vi "Frontend FPP_vdp_Ian_modified.vi"() -> ()   [LabVIEW 2016]
panel:
  in  "Gate 2":T1={"Gate Start"=0.0, "Gate Stop"=2.0, "Gate Step (linear only)"=1.0, "Gate Compliance"=0.0001, "Gate PComp"=0.0, "Range mode"=0, "Range"=6} {"Range" max=11 scale=0.0..11.0; "Range mode" items=["Auto", "Limited", "Fixed"]; "Gate PComp" format="%^.2e"; "Gate Compliance" format="%^.2e"; "Gate Step (linear only)" format="%^.4e"; "Gate Stop" format="%^.4e"; "Gate Start" format="%^.4e"}
  in  "Drain":T2={"Drain Start"=0.0, "Drain Stop"=2.0, "Drain Compliance"=0.0001, "Drain Step"=1.0, "Drain PComp"=0.0, "Range mode"=0, "Range"=6} {"Range" max=11 scale=0.0..11.0; "Range mode" items=["Auto", "Limited", "Fixed"]; "Drain PComp" format="%^.2e"; "Drain Step" format="%^.4e"; "Drain Compliance" format="%^.2e"; "Drain Stop" format="%^.4e"; "Drain Start" format="%^.4e"}
  in  "Gate":T3={"Gate Start"=0.0, "Gate Stop"=2.0, "Gate Step"=1.0, "Gate Compliance"=0.0001, "Gate PComp"=0.0, "Range mode"=0, "Range"=6} {"Range" max=11 scale=0.0..11.0; "Range mode" items=["Auto", "Limited", "Fixed"]; "Gate PComp" format="%^.2e"; "Gate Compliance" format="%^.2e"; "Gate Step" format="%^.4e"; "Gate Stop" format="%^.4e"; "Gate Start" format="%^.4e"}
  in  "Drain 2":T4={"Drain Start"=0.0, "Drain Stop"=2.0, "Drain Compliance"=0.0001, "Drain Step (linear only)"=1.0, "Drain PComp"=0.0, "Range mode"=0, "Range"=6} {"Range" max=11 scale=0.0..11.0; "Range mode" items=["Auto", "Limited", "Fixed"]; "Drain PComp" format="%^.2e"; "Drain Step (linear only)" format="%^.4e"; "Drain Compliance" format="%^.2e"; "Drain Stop" format="%^.4e"; "Drain Start" format="%^.4e"}
  in  "Timings":T5={"integration time"=0, "Short/Long integration time"=0.00064, "hold time (sec)"=0.0, "delay time (sec)"=0.0, "Step Time (0 disables)"=0.0, "sweep method"=0, "Pulse period"=0.005, "Base voltage"=0.0, "Pulse width"=0.0005} {"Pulse width" min=0.0005 max=0.1 step=0.0001 format="%.4f"; "Base voltage" format="%^.4e"; "Pulse period" min=0.005 max=1.0 step=0.0001 format="%.4f"; "sweep method" items=["Continuous", "Pulsed"]; "Step Time (0 disables)" format="%.2f"; "delay time (sec)" format="%.4f"; "hold time (sec)" format="%.4f"; "Short/Long integration time" format="%^.0e"; "integration time" scale=0.0..2.0}
  in  "Panel controls":T6={"Emergency Stop"=refnum, "OutputGraph Max"=1e-05, "Text/Graph (text=false)"=FALSE} {"OutputGraph Max" format="%.2e"}
  in  "Panel Controls":T7={"Emergency Stop"=refnum, "TransGraph Max"=1e-05, "Text/Graph (text=false)"=FALSE} {"TransGraph Max" format="%.2e"}
  in  "Tab Control":enum32{"Characteristics", "Other parameters"}(tab)
  in  "Van der Pauw":bool
  out "XY Graph 2":cluster{"Y data in":dbl[], "X data in":dbl[]}[](graph)
  in  "Integration time (long)":dbl=0.32 min=0.04 max=2.0 step=0.02 format="%.2f"
  in  "Integration time (short)":dbl=0.00064 min=8e-05 max=0.00192 step=8e-05 format="%^.0e"
  in  "Drain Range":u8(slide)=6 max=11 scale=0.0..11.0
  in  "Drain Range mode":u16(ring) items=["Auto", "Limited", "Fixed"]
  in  "Gate Range":u8(slide)=6 max=11 scale=0.0..11.0
  in  "Gate Range mode":u16(ring) items=["Auto", "Limited", "Fixed"]
  in  "Sampling mode":u32(slide) scale=0.0..4.0
  in  "Number of Samples":i32=500 min=0 step=1
  in  "Time":dbl=240.0 min=0.0 format="%.2f"
  in  "Drain":dbl=-10.0 min=-100.0 max=100.0 format="%.2f"
  in  "Gate":dbl=-60.0 min=-100.0 max=100.0 format="%.2f"
  in  "sweep method":u16(ring) items=["Continuous", "Pulsed"]
  out "Id":dbl format="%.2e"
  out "Ig":dbl format="%.2e"
  in  "Sweep Start":bool caption="Sweep start"
  in  "Interrupt run":bool
  in  "Running":bool
  out "Path":path
  in  "integration time":u32(slide)=1 max=2 step=1 scale=0.0..2.0
  in  "sweep mode":u16(ring)=1 items=["Single", "Double"]
  in  "Transfer Start":bool
  in  "Output Start":bool
  in  "Drain: Step":dbl=-0.1 min=-100.0 max=100.0 format="%.2f"
  in  "Drain: Stop":dbl=-1.0 min=-100.0 max=100.0 format="%.2f"
  in  "Drain:Start":dbl=1.0 min=-100.0 max=100.0 format="%.2f"
  in  "Gate: Step":dbl min=-100.0 max=100.0 format="%.2f"
  in  "Gate: Stop":dbl min=-100.0 max=100.0 format="%.2f"
  in  "Gate: Start":dbl min=-100.0 max=100.0 format="%.2f"
  out "XY Graph":cluster{"Y data in":dbl[], "X data in":dbl[]}[](graph)
  in  "Drain: Compliance":dbl=0.001 min=1e-12 max=0.02 format="%.8f"
  in  "Gate: Compliance":dbl=0.001 min=1e-12 max=0.02 format="%.8f"
  in  "Drain: Step":dbl=-5.0 min=-100.0 max=100.0 format="%.2f"
  in  "Drain: Stop":dbl=-10.0 min=-100.0 max=100.0 format="%.2f"
  in  "Drain:Start":dbl=-5.0 min=-100.0 max=100.0 format="%.2f"
  in  "Gate: Step":dbl=-1.0 min=-100.0 max=100.0 format="%.2f"
  in  "Gate: Stop":dbl=-60.0 min=-100.0 max=100.0 format="%.2f"
  in  "Gate: Start":dbl=10.0 min=-100.0 max=100.0 format="%.2f"
  out "Vp_2":dbl format="%.2e"
  out "Vp_1":dbl format="%.2e"
  out "Delta V":dbl format="%.2e"
  out "Conductivity (S/cm)":dbl format="%.2e"
  in  "Thickness (m)":dbl=4e-08 min=1e-09 max=100.0 format="%.2e"
  in  "Hall Bar Channel Length  (L in m)":dbl=2e-05 format="%#_13g"
  in  "Hall Bar Channel Width (W in m)":dbl=4e-05 format="%#_13g"
  in  "Pulse width":dbl=0.0005 min=0.0005 max=0.1 step=0.0001 format="%.4f"
  in  "Base voltage":dbl min=-100.0 max=100.0 format="%.2f"
  in  "Pulse period":dbl=0.005 min=0.005 max=1.0 step=0.0001 format="%.4f"
  in  "Drain Power Compliance":dbl min=0.0 max=1.0 format="%.2f"
  in  "Gate Power\nCompliance":dbl min=0.0 max=1.0 format="%.2f"
  in  "OutputGraph Max":dbl=1e-05 format="%.2e"
  in  "TransGraph Max":dbl=1e-05 format="%.2e"
  in  "SPA Display":bool
  in  "Step delay /s":dbl min=0.0 max=1.0 format="%.2f"
  in  "hold time /s":dbl min=0.0 max=655.35 step=0.01 format="%.2f"
  in  "delay time /s":dbl min=0.0 max=65.535 step=0.0001 format="%.2f"
  in  "Decimal places in header":i8=1
  out "error out":errorcluster
  # "Transfer Characteristics"
  # "Stress Measurements"
  # "V"
  # "V"
  # "V"
  # "Gate"
  # "V"
  # "V"
  # "V"
  # "V"
  # "Drain"
  # "V"
  # "Output Characteristics"
  # "s"
  # "V"
  # "V"
  # "V"
  # "Gate"
  # "V"
  # "V"
  # "Drain"
  # "V"
  # "For Four Point Probe measurements ONLY!"
  # "SMU1 = Probe 1\nSMU2 = Drain\nSMU3 = Gate\nSMU4 = Probe 2\nVSU1 = Source"
  # "A"
  # "A"
  # "Vp1"
  # "Vp2"
  # "s"
  # "Pulsed mode settings"
  # "s"
  # "NOTE - THIS OVERRIDES THE COMPLIANCE VALUES!"
  # "A"
  # "A"
  # "Enter max power in Watts (max 1W)"
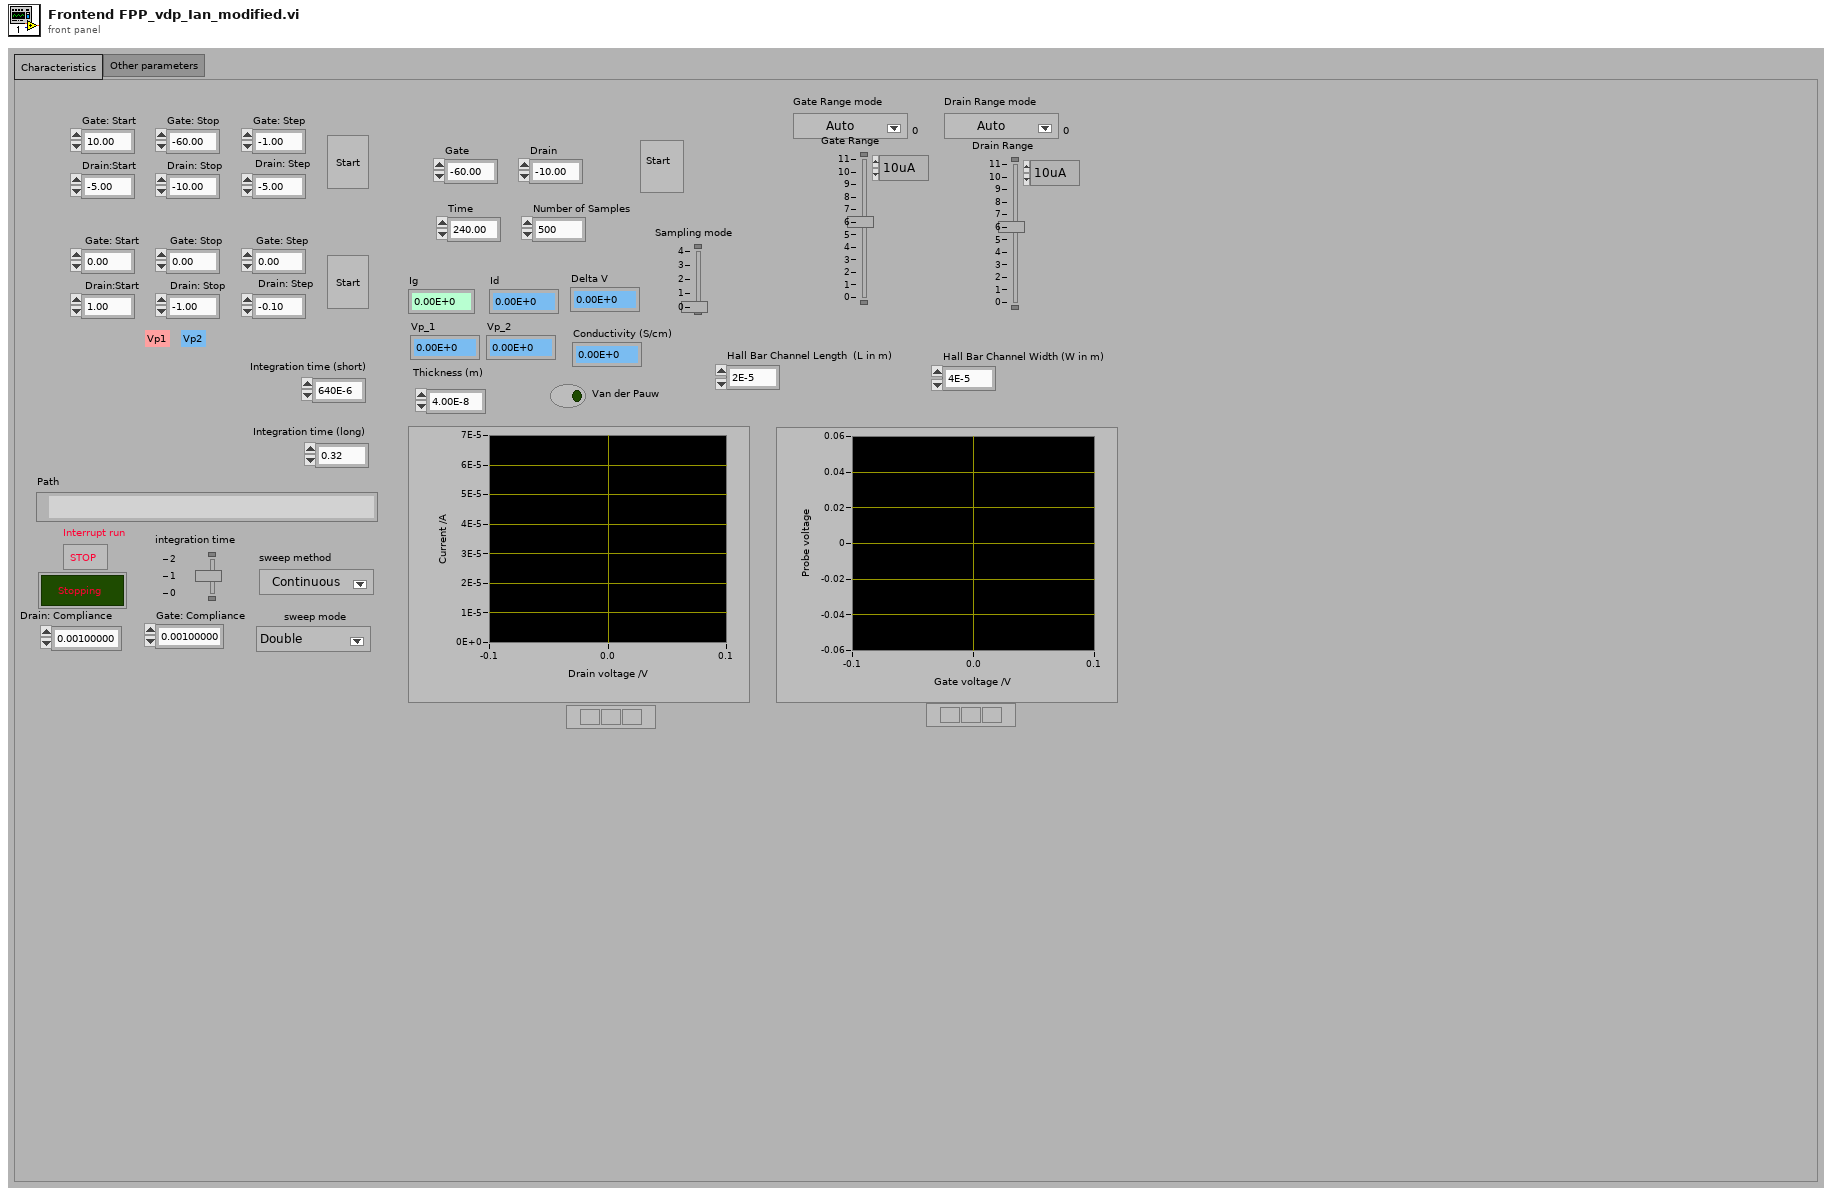
[diagram p1: front panel]
types:
  T1 = cluster{"Gate Start":dbl, "Gate Stop":dbl, "Gate Step (linear only)":dbl, "Gate Compliance":dbl, "Gate PComp":dbl, "Range mode":u16, "Range":u8}
  T2 = cluster{"Drain Start":dbl, "Drain Stop":dbl, "Drain Compliance":dbl, "Drain Step":dbl, "Drain PComp":dbl, "Range mode":u16, "Range":u8}
  T3 = cluster{"Gate Start":dbl, "Gate Stop":dbl, "Gate Step":dbl, "Gate Compliance":dbl, "Gate PComp":dbl, "Range mode":u16, "Range":u8}
  T4 = cluster{"Drain Start":dbl, "Drain Stop":dbl, "Drain Compliance":dbl, "Drain Step (linear only)":dbl, "Drain PComp":dbl, "Range mode":u16, "Range":u8}
  T5 = cluster{"integration time":u32, "Short/Long integration time":dbl, "hold time (sec)":dbl, "delay time (sec)":dbl, "Step Time (0 disables)":dbl, "sweep method":u16, "Pulse period":dbl, "Base voltage":dbl, "Pulse width":dbl}
  T6 = cluster{"Emergency Stop":refnum<vi>, "OutputGraph Max":dbl, "Text/Graph (text=false)":bool}
  T7 = cluster{"Emergency Stop":refnum<vi>, "TransGraph Max":dbl, "Text/Graph (text=false)":bool}
  T8 = cluster{"V2 Start":dbl, "V2 Step":dbl, "Number of points":i32}
  T9 = enum16{"open", "replace", "create", "open or create", "replace or create", "replace or create with confirmation"}
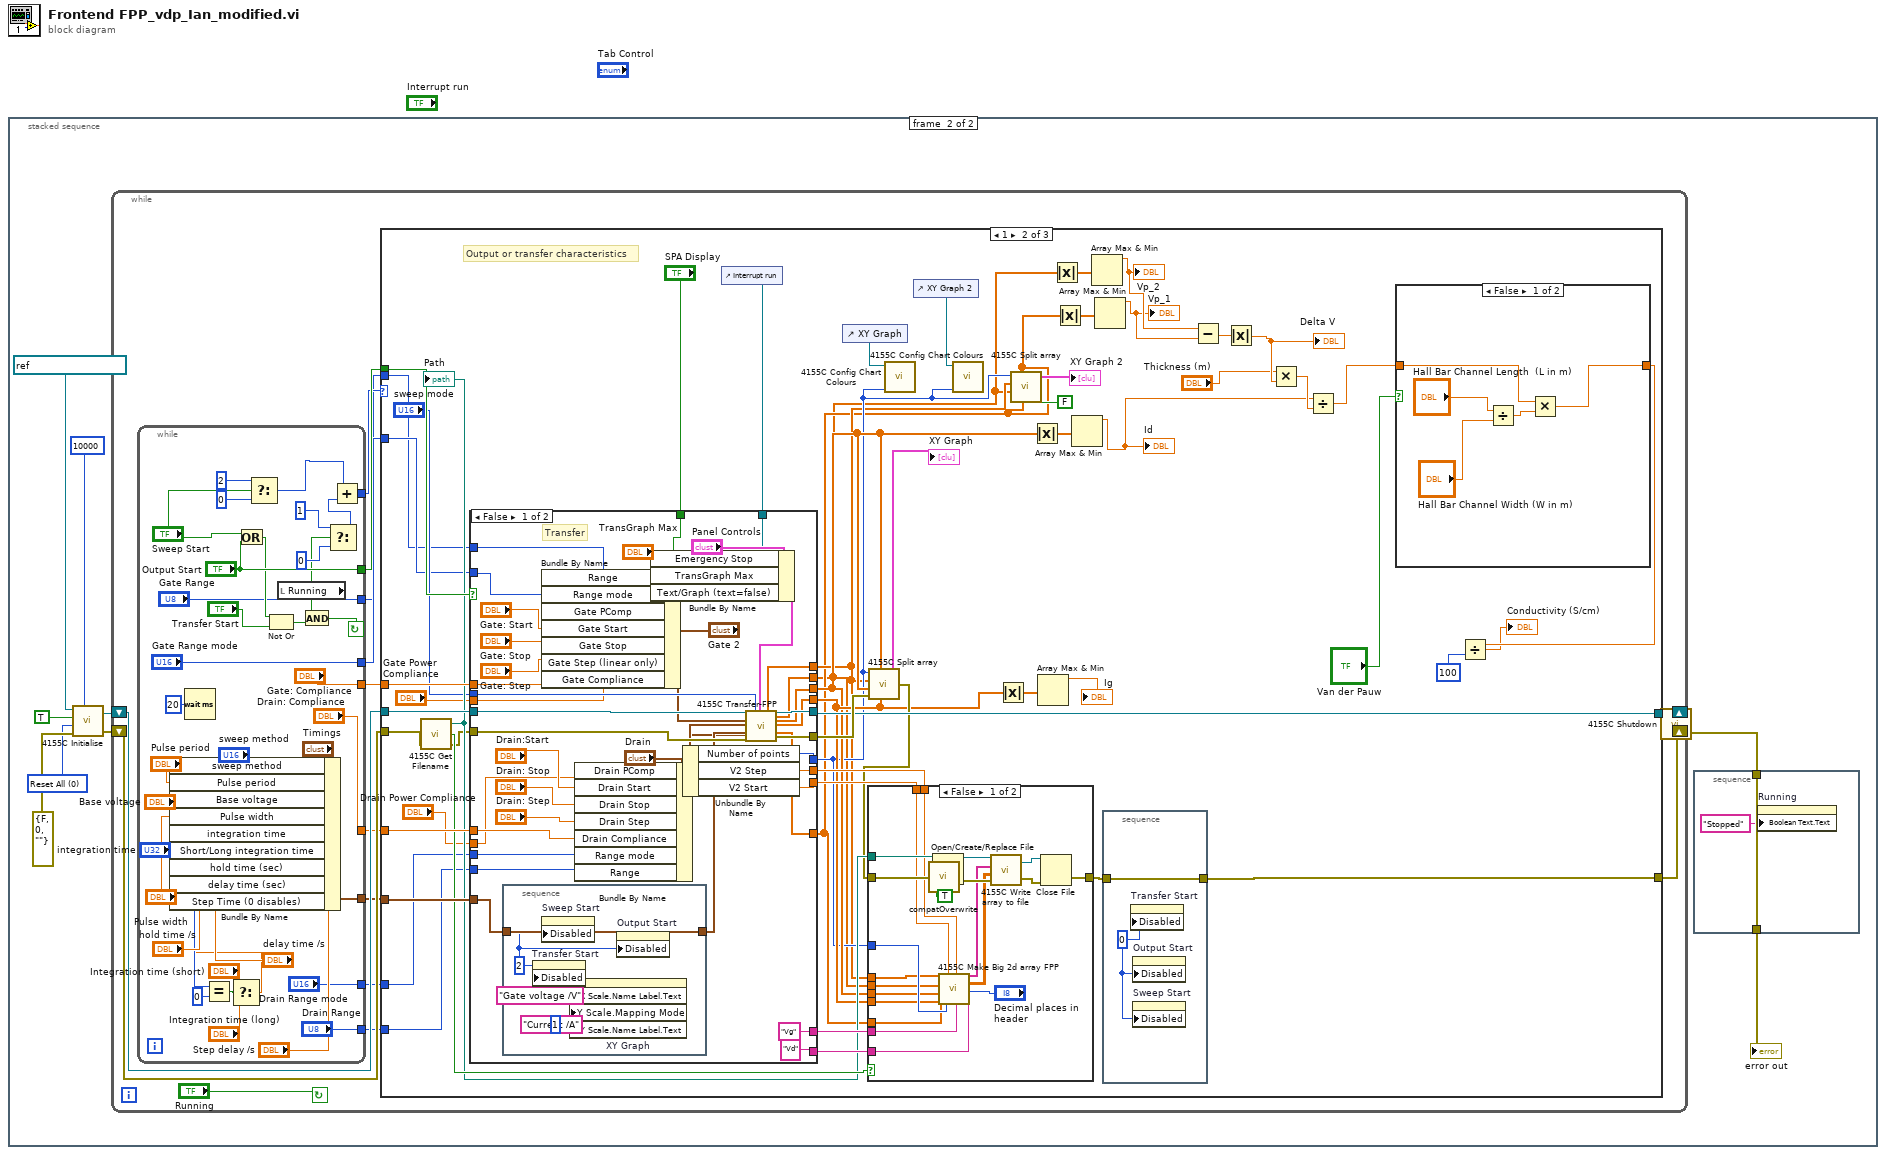
[diagram p0: block diagram]
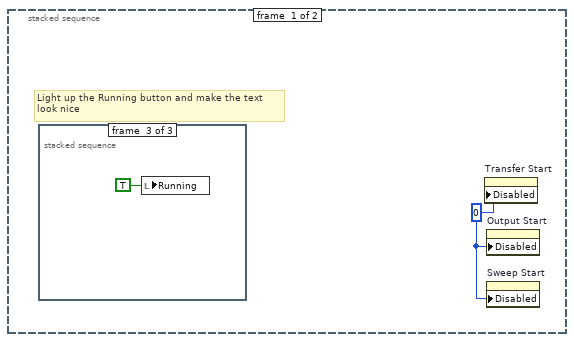
[diagram p2: hidden frame]
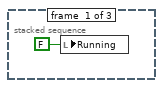
[diagram p3: hidden frame]
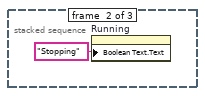
[diagram p4: hidden frame]
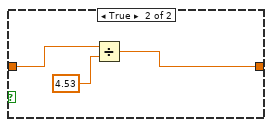
[diagram p6: hidden frame]
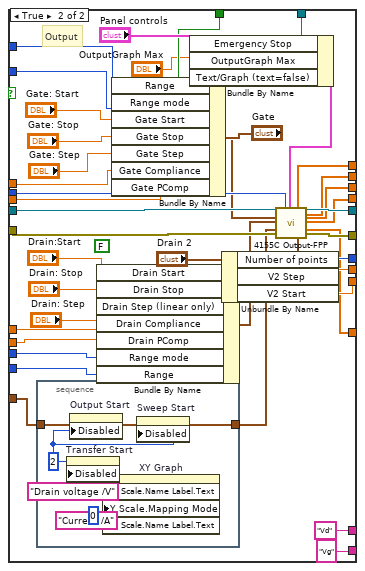
[diagram p8: hidden frame]
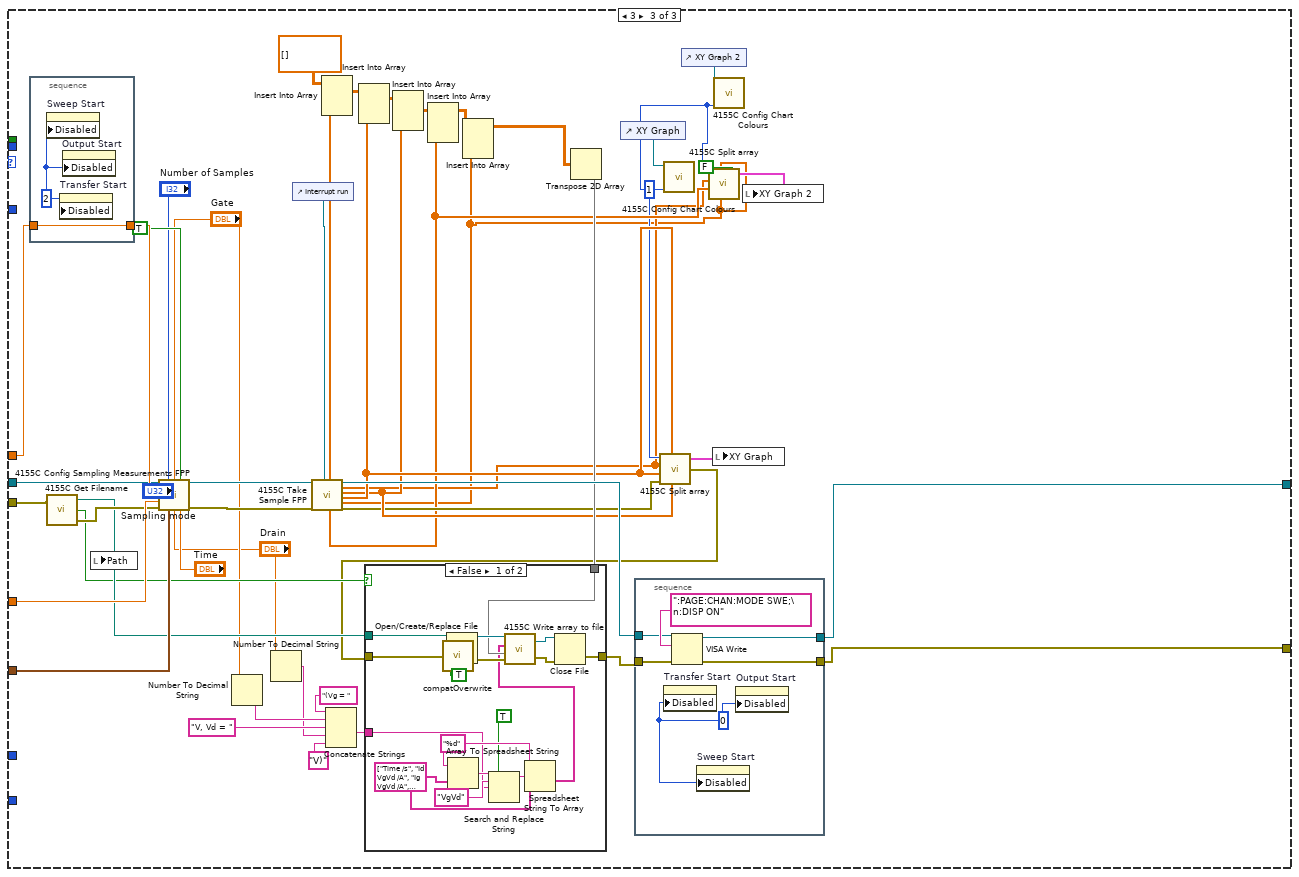
[diagram p9: hidden frame]
diagram:
  n1 = stacked-sequence {
    frame #0 {
      w1 = u8 0 ("Disabled")
      # "Light up the Running button and make the text\nlook nice"
      n2 = stacked-sequence {
        frame #0 {
          n3 = local write "Running"(FALSE ("Running")) -> ()
        }
        frame #1 {
          n4 = property on="Running" class="Bool (strict)"("Boolean Text.Text"="Stopping") -> ()  [unwired: 2 in, 2 out]
        }
        frame #2 {
          (unwired) FALSE ("Running")
          n5 = local write "Running"(TRUE ("Running")) -> ()
        }
      }
      n6 = property on="Transfer Start" class="Bool (strict)"("Disabled"=w1) -> ()  [unwired: 2 in, 2 out]
      n7 = property on="Output Start" class="Bool (strict)"("Disabled"=w1) -> ()  [unwired: 2 in, 2 out]
      n8 = property on="Sweep Start" class="Bool (strict)"("Disabled"=w1) -> ()  [unwired: 2 in, 2 out]
    }
    frame #1 {
      w11 = u16 0 items=["Reset All", "Partial reset"] ("Type of reset")
      n9 = call "4155C Initialise.vi"("VISA resource name in"=refnum<visa-resource-name> "GPIB0::14::INSTR", "Reset"=TRUE, "Type of reset"=w11, "error in (no error)"=errorcluster {"status"=FALSE, "code"=0, "source"=""}, "VISA Timeout Value"=u32 10000) -> ("VISA Resource Name out"=w10:refnum<visa-resource-name>, "error out"=w9:errorcluster)
      n10 = while {
        shift-left: w10 -> [w24]
        shift-right: [w26] -> w5
        shift-left: w9 -> [w25]
        shift-right: [w27] -> w6
        stop <- "Running" continue-if-true
        n11 = while {
          tunnel: ["Gate Range"] -> w16
          tunnel: ["Gate Range mode"] -> w17
          tunnel: ["Drain Range"] -> w18
          tunnel: ["Drain Range mode"] -> w19
          tunnel: ["Drain: Compliance"] -> w20
          tunnel: [w49] -> w21
          tunnel: ["Gate: Compliance"] -> w22
          tunnel: [w55] -> w23
          tunnel: ["Output Start"] -> w28
          stop <- w64 continue-if-true
          n12 = Wait (ms)(milliseconds to wait=u32 20) -> ()  [unwired: 1 out]
          n13 = Equal?(x="integration time", y=u32 0) -> (x = y?=w46:bool)
          n14 = Select(t="Integration time (short)", s=w46, f="Integration time (long)") -> (s? t:f=w43:dbl)
          n15 = Bundle By Name(cluster="Timings", "sweep method"="sweep method", "Pulse period"="Pulse period", "Base voltage"="Base voltage", "Pulse width"="Pulse width", "integration time"="integration time", "Short/Long integration time"=w43, "hold time (sec)"="hold time /s", "delay time (sec)"="delay time /s", "Step Time (0 disables)"="Step delay /s") -> (w49:T5)
          n16 = Or(x="Sweep Start", y="Output Start") -> (x .or. y?=w61:bool)
          n17 = Select(t=i8 2, s="Sweep Start", f=i8 0) -> (s? t:f=w31:i8)
          n18 = Not Or(1:"Transfer Start", 2:w61) -> (0:w63:bool)
          n19 = local read "Running"() -> (w58:bool)
          n20 = And(x=w58, y=w63) -> (x .and. y?=w64:bool)
          n21 = Select(t=i8 1, s=w58, f=i8 0) -> (s? t:f=w54:i8)
          n22 = Add(x=w31, y=w54) -> (x+y=w55:i8)
        }
        n23 = case shown="1" w23 {
          tunnel: w28 -> [_ w122 _]
          tunnel: w21 -> [_ w121 w287]
          tunnel: w22 -> [_ w120 w295]
          tunnel: w20 -> [_ w119 w291]
          tunnel: [w67 w110 w293] -> w27
          tunnel: [w66 w113 w294] -> w26
          tunnel: w25 -> [w67 w104 w282]
          tunnel: w24 -> [w66 w112 w281]
          tunnel: w19 -> [_ w94 _]
          tunnel: w18 -> [_ w93 _]
          tunnel: w17 -> [_ w92 _]
          tunnel: w16 -> [_ w91 _]
          frame 0, Default {
            # "Someone's deselected the running button so just shutdown..."
          }
          frame 1 {
            # "Output or transfer characteristics"
            n24 = call "4155C Get Filename.vi"("error in (no error)"=w104) -> ("error out"=w103:errorcluster, "cancelled"=w109:bool, "path"=w108:path)  [unwired: 2 in]
            "Path" <- w108
            n25 = control-ref of="Interrupt run"() -> (w105:refnum<vi>)
            n26 = case shown="False" w122 {
              tunnel: w112 -> [w182 w228]
              tunnel: w103 -> [w181 w227]
              tunnel: w121 -> [w185 w233]
              tunnel: w120 -> [w191 w240]
              tunnel: w119 -> [w196 w239]
              tunnel: "sweep mode" -> [w190 w238]
              tunnel: [w158 w206] -> w85
              tunnel: [w157 w205] -> w80
              tunnel: [w160 w204] -> w90
              tunnel: [w159 w203] -> w95
              tunnel: [w189 w237] -> w113
              tunnel: [w188 w236] -> w118
              tunnel: [w161 w209] -> w86
              tunnel: [w162 w208] -> w116
              tunnel: [w163 w207] -> w117
              tunnel: ["Vg" "Vd"] -> w115
              tunnel: ["Vd" "Vg"] -> w114
              tunnel: w105 -> [w179 w226]
              tunnel: "SPA Display" -> [w178 w224]
              tunnel: "Drain Power Compliance" -> [w174 w221]
              tunnel: "Gate Power\nCompliance" -> [w175 w220]
              tunnel: w94 -> [w166 w214]
              tunnel: w93 -> [w165 w213]
              tunnel: w92 -> [w167 w212]
              tunnel: w91 -> [w168 w211]
              tunnel: [w156 w202] -> w82
              frame False {
                # "Transfer"
                n27 = stacked-sequence {
                  tunnel: w185 -> [w200]
                  tunnel: [w200] -> w173
                  frame #0 {
                    w198 = u8 2 ("Disabled")
                    n28 = property on="Transfer Start" class="Bool (strict)"("Disabled"=w198) -> ()  [unwired: 2 in, 2 out]
                    n29 = property on="Sweep Start" class="Bool (strict)"("Disabled"=w198) -> ()  [unwired: 2 in, 2 out]
                    n30 = property on="XY Graph" class="XYGraph (strict)"("X Scale.Name Label.Text"="Gate voltage /V", "Y Scale.Mapping Mode"=u8 1, "Y Scale.Name Label.Text"="Current /A") -> ()  [unwired: 2 in, 2 out]
                    n31 = property on="Output Start" class="Bool (strict)"("Disabled"=w198) -> ()  [unwired: 2 in, 2 out]
                  }
                }
                n32 = Bundle By Name(cluster="Gate 2", "Range"=w168, "Range mode"=w167, "Gate PComp"=w175, "Gate Start"="Gate: Start", "Gate Stop"="Gate: Stop", "Gate Step (linear only)"="Gate: Step", "Gate Compliance"=w191) -> (w169:T1)
                n33 = Bundle By Name(cluster="Drain", "Drain PComp"=w174, "Drain Start"="Drain:Start", "Drain Stop"="Drain: Stop", "Drain Step"="Drain: Step", "Drain Compliance"=w196, "Range mode"=w166, "Range"=w165) -> (w171:T2)
                n34 = Bundle By Name(cluster="Panel Controls", "Emergency Stop"=w179, "TransGraph Max"="TransGraph Max", "Text/Graph (text=false)"=w178) -> (w176:T7)
                n35 = call "4155C Transfer-FPP.vi"("VISA resource name in"=w182, "Gate"=w169, "Drain"=w171, "Timings"=w173, "error in (no error)"=w181, "sweep mode"=w190, "Panel Controls"=w176) -> ("VG"=w158:dbl[], "Outparams"=w164:T8, "VISA Resource Name out"=w189:refnum<visa-resource-name>, "Vprobe2"=w157:dbl[], "ID"=w160:dbl[], "IG"=w159:dbl[], "Vprobe1"=w156:dbl[], "error out"=w188:errorcluster)  [unwired: 13 in]
                n36 = Unbundle By Name(w164) -> ("Number of points"=w161:i32, "V2 Step"=w162:dbl, "V2 Start"=w163:dbl)
              }
              frame True {
                (unwired) FALSE ("Logarithmic")
                # "Output"
                n37 = stacked-sequence {
                  tunnel: w233 -> [w246]
                  tunnel: [w246] -> w219
                  frame #0 {
                    w244 = u8 2 ("Disabled")
                    n38 = property on="Transfer Start" class="Bool (strict)"("Disabled"=w244) -> ()  [unwired: 2 in, 2 out]
                    n39 = property on="Output Start" class="Bool (strict)"("Disabled"=w244) -> ()  [unwired: 2 in, 2 out]
                    n40 = property on="XY Graph" class="XYGraph (strict)"("X Scale.Name Label.Text"="Drain voltage /V", "Y Scale.Mapping Mode"=u8 0, "Y Scale.Name Label.Text"="Current /A") -> ()  [unwired: 2 in, 2 out]
                    n41 = property on="Sweep Start" class="Bool (strict)"("Disabled"=w244) -> ()  [unwired: 2 in, 2 out]
                  }
                }
                n42 = Bundle By Name(cluster="Drain 2", "Drain Start"="Drain:Start", "Drain Stop"="Drain: Stop", "Drain Step (linear only)"="Drain: Step", "Drain Compliance"=w239, "Drain PComp"=w221, "Range mode"=w214, "Range"=w213) -> (w217:T4)
                n43 = Bundle By Name(cluster="Gate", "Range"=w211, "Range mode"=w212, "Gate Start"="Gate: Start", "Gate Stop"="Gate: Stop", "Gate Step"="Gate: Step", "Gate Compliance"=w240, "Gate PComp"=w220) -> (w215:T3)
                n44 = Bundle By Name(cluster="Panel controls", "Emergency Stop"=w226, "OutputGraph Max"="OutputGraph Max", "Text/Graph (text=false)"=w224) -> (w222:T6)
                n45 = call "4155C Output-FPP.vi"("VISA resource name in"=w228, "Gate"=w215, "Drain"=w217, "Timings"=w219, "error in (no error)"=w227, "sweep mode"=w238, "Panel controls"=w222) -> ("VD"=w206:dbl[], "Outparams"=w210:T8, "VISA Resource Name out"=w237:refnum<visa-resource-name>, "Vprobe2"=w205:dbl[], "ID"=w204:dbl[], "IG"=w203:dbl[], "Vprobe1"=w202:dbl[], "error out"=w236:errorcluster)  [unwired: 13 in]
                n46 = Unbundle By Name(w210) -> ("Number of points"=w209:i32, "V2 Step"=w208:dbl, "V2 Start"=w207:dbl)
              }
            }
            n47 = control-ref of="XY Graph"() -> (w106:refnum<vi>)
            n48 = call "4155C Split array.vi"("Number of VAR2 steps"=w86, "Y2 data in"=w90, "X data in"=w85, "Y1 data in"=w90, "Y3 data in"=w95, "error in (no error)"=w118) -> ("Array of clusters"=→"XY Graph":cluster{"Y data in":dbl[], "X data in":dbl[]}[], "error out"=w102:errorcluster)  [unwired: 1 in]
            n49 = case shown="False" w109 {
              tunnel: w102 -> [w153 w155]
              tunnel: [w148 w155] -> w111
              tunnel: w108 -> [w152 _]
              tunnel: w86 -> [w146 _]
              tunnel: w90 -> [w136 _]
              tunnel: w85 -> [w138 _]
              tunnel: w80 -> [w137 _]
              tunnel: w95 -> [w135 _]
              tunnel: w117 -> [w140 _]
              tunnel: w116 -> [w141 _]
              tunnel: w115 -> [w145 _]
              tunnel: w114 -> [w144 _]
              tunnel: w82 -> [w134 _]
              frame False {
                n50 = call <vilib>:"compatOverwrite.vi"("overwrite (F)"=TRUE) -> ("overwrite?"=w133:T9)
                n51 = Open/Create/Replace File(file path (use dialog)=w152, error in=w153, operation (0:open)=w133) -> (refnum out=w150:refnum<file>, error out=w151:errorcluster)  [unwired: 3 in, 1 out]
                n52 = call "4155C Make Big 2d array FPP.vi"("1D Var1"=w138, "1d ID"=w136, "1d Vp2"=w137, "1d IG"=w135, "1d Vp1"=w134, "VAR2 START"=w140, "Number of VAR2 steps"=w146, "VAR2 STEP"=w141, "VAR1 Name"=w145, "Decimal places in header"="Decimal places in header", "VAR2 Name"=w144) -> ("Header array"=w142:string[], "Data array"=w143:dbl[][])  [unwired: 15 in]
                n53 = call "4155C Write array to file.vi"("Byte Stream File Refnum"=w150, "Header"=w142, "Data Array"=w143, "error in (no error)"=w151) -> ("dup refnum"=w147:refnum<file>, "error out"=w149:errorcluster)  [unwired: 1 in]
                n54 = Close File(refnum=w147, error in=w149) -> (error out=w148:errorcluster)  [unwired: 1 out]
              }
              frame True {
              }
            }
            n55 = call "4155C Config Chart Colours.vi"("Numeric"=w86, "XY Graph 2"=w106) -> ()  [unwired: 6 in]
            n56 = control-ref of="XY Graph 2"() -> (w88:refnum<vi>)
            n57 = call "4155C Config Chart Colours.vi"("Numeric"=w86, "XY Graph 2"=w88) -> ()  [unwired: 6 in]
            n58 = Absolute Value(x=w95) -> (abs(x)=w97:dbl[])
            n59 = call "4155C Split array.vi"("Number of VAR2 steps"=w86, "Y2 data in"=w82, "X data in"=w85, "Y1 data in"=w80, "Y3 data in"=w82, "Absolute val?"=FALSE) -> ("Array of clusters"=→"XY Graph 2":cluster{"Y data in":dbl[], "X data in":dbl[]}[])  [unwired: 1 in, 1 out]
            n60 = Absolute Value(x=w90) -> (abs(x)=w96:dbl[])
            n61 = Array Max & Min(array=w97) -> (max value=→"Ig":dbl)  [unwired: 3 out]
            n62 = Absolute Value(x=w80) -> (abs(x)=w81:dbl[])
            n63 = Absolute Value(x=w82) -> (abs(x)=w83:dbl[])
            n64 = Array Max & Min(array=w96) -> (max value=w71:dbl)  [unwired: 3 out]
            "Id" <- w71
            n65 = Array Max & Min(array=w81) -> (max value=w79:dbl)  [unwired: 3 out]
            "Vp_2" <- w79
            n66 = Array Max & Min(array=w83) -> (max value=w78:dbl)  [unwired: 3 out]
            "Vp_1" <- w78
            n67 = stacked-sequence {
              tunnel: w111 -> [w132]
              tunnel: [w132] -> w110
              frame #0 {
                w131 = u8 0 ("Disabled")
                n68 = property on="Transfer Start" class="Bool (strict)"("Disabled"=w131) -> ()  [unwired: 2 in, 2 out]
                n69 = property on="Output Start" class="Bool (strict)"("Disabled"=w131) -> ()  [unwired: 2 in, 2 out]
                n70 = property on="Sweep Start" class="Bool (strict)"("Disabled"=w131) -> ()  [unwired: 2 in, 2 out]
              }
            }
            n71 = Subtract(x=w79, y=w78) -> (x-y=w77:dbl)
            n72 = Absolute Value(x=w77) -> (abs(x)=w76:dbl)
            "Delta V" <- w76
            n73 = Multiply(x="Thickness (m)", y=w76) -> (x*y=w72:dbl)
            n74 = Divide(x=w71, y=w72) -> (x/y=w73:dbl)
            n75 = case shown="False" "Van der Pauw" {
              tunnel: [w125 w129] -> w70
              tunnel: w73 -> [w126 w130]
              frame False {
                n76 = Divide(x="Hall Bar Channel Length  (L in m)", y="Hall Bar Channel Width (W in m)") -> (x/y=w127:dbl)
                n77 = Multiply(x=w126, y=w127) -> (x*y=w125:dbl)
              }
              frame True {
                n78 = Divide(x=w130, y=4.53) -> (x/y=w129:dbl)
              }
            }
            n79 = Divide(x=w70, y=100) -> (x/y=→"Conductivity (S/cm)":dbl)
          }
          frame 3 {
            w251 = 1 ("Numeric")
            n80 = stacked-sequence {
              tunnel: w295 -> [w322]
              tunnel: [w322] -> w292
              frame #0 {
                w321 = u8 2 ("Disabled")
                n81 = property on="Sweep Start" class="Bool (strict)"("Disabled"=w321) -> ()  [unwired: 2 in, 2 out]
                n82 = property on="Transfer Start" class="Bool (strict)"("Disabled"=w321) -> ()  [unwired: 2 in, 2 out]
                n83 = property on="Output Start" class="Bool (strict)"("Disabled"=w321) -> ()  [unwired: 2 in, 2 out]
              }
            }
            n84 = call "4155C Get Filename.vi"("error in (no error)"=w282) -> ("error out"=w280:errorcluster, "cancelled"=w271:bool, "path"=w272:path)  [unwired: 2 in]
            n85 = local write "Path"(w272) -> ()
            n86 = call "4155C Config Sampling Measurements FPP.vi"("VISA session"=w281, "Num Points"="Number of Samples", "Vg"="Gate", "Display on/off"=TRUE, "Gate Compliance"=w292, "Sampling mode"="Sampling mode", "Drain Compliance"=w291, "error in (no error)"=w280, "Timings"=w287, "Vd"="Drain", "Sample time"="Time") -> ("dup VISA resource name"=w288:refnum<visa-resource-name>, "error out"=w289:errorcluster)  [unwired: 3 in]
            n87 = Number To Decimal String(number="Gate") -> (decimal integer string=w269:string)  [unwired: 1 in]
            n88 = Number To Decimal String(number="Drain") -> (decimal integer string=w267:string)  [unwired: 1 in]
            n89 = control-ref of="Interrupt run"() -> (w283:refnum<vi>)
            n90 = call "4155C Take Sample FPP.vi"("VISA resource name in"=w288, "error in (no error)"=w289, "Emergency Stop"=w283) -> ("Time"=w249:dbl[], "Vp1"=w253:dbl[], "VISA Resource Name out"=w290:refnum<visa-resource-name>, "Ig"=w261:dbl[], "Id"=w262:dbl[], "Vp2"=w248:dbl[], "error out"=w260:errorcluster)  [unwired: 10 in]
            n91 = Insert Into Array(array=dbl[][] [] ("Input Array"), new element=w249) -> (w279:dbl[][])  [unwired: 2 in]
            n92 = Concatenate Strings("(Vg = " ("Substring"), w269, "V, Vd = " ("Substring"), w267, "V)" ("Substring")) -> (w265:string)
            n93 = Insert Into Array(array=w279, new element=w262) -> (w278:dbl[][])  [unwired: 2 in]
            n94 = Insert Into Array(array=w278, new element=w261) -> (w277:dbl[][])  [unwired: 2 in]
            n95 = Insert Into Array(array=w277, new element=w253) -> (w275:dbl[][])  [unwired: 2 in]
            n96 = Insert Into Array(array=w275, new element=w248) -> (w255:dbl[][])  [unwired: 2 in]
            n97 = Transpose 2D Array(2D array=w255) -> (transposed array=w273:dbl[][])
            n98 = control-ref of="XY Graph"() -> (w264:refnum<vi>)
            n99 = call "4155C Split array.vi"("Number of VAR2 steps"=w251, "Y2 data in"=w262, "X data in"=w249, "Y1 data in"=w262, "Y3 data in"=w261, "error in (no error)"=w260) -> ("Array of clusters"=w263:cluster{"Y data in":dbl[], "X data in":dbl[]}[], "error out"=w259:errorcluster)  [unwired: 1 in]
            n100 = case shown="False" w271 {
              tunnel: w259 -> [w312 w314]
              tunnel: [w307 w314] -> w274
              tunnel: w272 -> [w311 _]
              tunnel: w273 -> [w305 _]
              tunnel: w265 -> [w297 _]
              frame False {
                w298 = string[] ["Time /s", "Id VgVd /A", "Ig VgVd /A", "Vp1 VgVd /V", "Vp2 VgVd /V"] ("Header")
                w302 = "%d" ("format string")
                n101 = call <vilib>:"compatOverwrite.vi"("overwrite (F)"=TRUE) -> ("overwrite?"=w296:T9)
                n102 = Open/Create/Replace File(file path (use dialog)=w311, error in=w312, operation (0:open)=w296) -> (refnum out=w309:refnum<file>, error out=w310:errorcluster)  [unwired: 3 in, 1 out]
                n103 = Array To Spreadsheet String(array=w298, 3:w302) -> (spreadsheet string=w304:string)  [unwired: 1 in]
                n104 = Search and Replace String(replace all?=TRUE ("replace all? (F)"), input string=w304, search string="VgVd", replace string=w297) -> (result string=w300:string)  [unwired: 4 in, 3 out]
                n105 = Spreadsheet String To Array(format string=w302, spreadsheet string=w300, array type (2D Dbl)=w298) -> (array=w299:string[])  [unwired: 1 in]
                n106 = call "4155C Write array to file.vi"("Byte Stream File Refnum"=w309, "Header"=w299, "Data Array"=w305, "error in (no error)"=w310) -> ("dup refnum"=w306:refnum<file>, "error out"=w308:errorcluster)  [unwired: 1 in]
                n107 = Close File(refnum=w306, error in=w308) -> (error out=w307:errorcluster)  [unwired: 1 out]
              }
              frame True {
              }
            }
            n108 = stacked-sequence {
              tunnel: [w317] -> w294
              tunnel: [w316] -> w293
              tunnel: w290 -> [w319]
              tunnel: w274 -> [w318]
              frame #0 {
                w315 = u8 0 ("Disabled")
                n109 = property on="Transfer Start" class="Bool (strict)"("Disabled"=w315) -> ()  [unwired: 2 in, 2 out]
                n110 = VISA Write(VISA resource name=w319, write buffer=":PAGE:CHAN:MODE SWE;\n:DISP ON" ("write buffer (\"\")"), error in (no error)=w318) -> (VISA resource name out=w317:refnum<visa-resource-name>, error out=w316:errorcluster)  [unwired: 1 out]
                n111 = property on="Sweep Start" class="Bool (strict)"("Disabled"=w315) -> ()  [unwired: 2 in, 2 out]
                n112 = property on="Output Start" class="Bool (strict)"("Disabled"=w315) -> ()  [unwired: 2 in, 2 out]
              }
            }
            n113 = call "4155C Config Chart Colours.vi"("Numeric"=w251, "XY Graph 2"=w264) -> ()  [unwired: 6 in]
            n114 = control-ref of="XY Graph 2"() -> (w254:refnum<vi>)
            n115 = call "4155C Split array.vi"("Number of VAR2 steps"=w251, "Y2 data in"=w248, "X data in"=w249, "Y1 data in"=w253, "Y3 data in"=w248, "Absolute val?"=FALSE) -> ("Array of clusters"=w252:cluster{"Y data in":dbl[], "X data in":dbl[]}[])  [unwired: 1 in, 1 out]
            n116 = local write "XY Graph"(w263) -> ()
            n117 = call "4155C Config Chart Colours.vi"("Numeric"=w251, "XY Graph 2"=w254) -> ()  [unwired: 6 in]
            n118 = local write "XY Graph 2"(w252) -> ()
          }
        }
      }
      n119 = call "4155C Shutdown.vi"("VISA resource name in"=w5, "error in (no error)"=w6) -> ("error out"=w8:errorcluster)  [unwired: 4 in]
      n120 = stacked-sequence {
        tunnel: w8 -> [w324]
        tunnel: [w324] -> w7
        frame #0 {
          n121 = property on="Running" class="Bool (strict)"("Boolean Text.Text"="Stopped") -> ()  [unwired: 2 in, 2 out]
        }
      }
      "error out" <- w7
    }
  }
